vi "Read any file DBL 1ch.vi"(6 "Data type":dbl[](array[numeric]), 7 "tdms file in":refnum<k34>, 8 "error in":errorcluster, 9 "Data File Type":T2(ring), 10 "Data window":T1={"Start"=0, "Length"=500000, "Channel numbers"=[0], "Channel name"="", "Group name"="Untitled"}, 11 "Input file path":path) -> (0 "error out":errorcluster, 1 "1st channel length":u64, 2 "Data out":dbl[](array[numeric]), 3 "Actual input file path":path, 4 "end of file?":bool, 5 "tdms file out":refnum<k34>)   [LabVIEW 2015]
uses:
  Data window.ctl
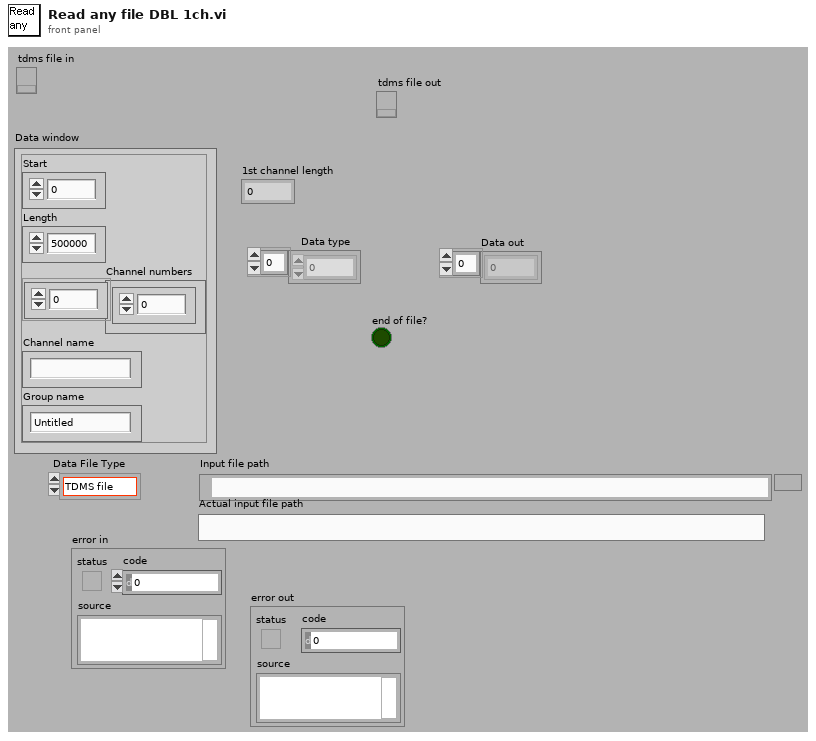
[diagram p1: front panel]
types:
  T1 = typedef "Data window.ctl" = cluster{"Start":i64, "Length":i32, "Channel numbers":i64[], "Channel name":string, "Group name":string}
  T2 = enum16{"TDMS file", "Tektronics ISF", "BinF file", "ASCII File", "BinH File", "BinW File", "BINARY File"}
  T3 = enum16{"open", "open or create", "create or replace", "create", "open (read-only)"}
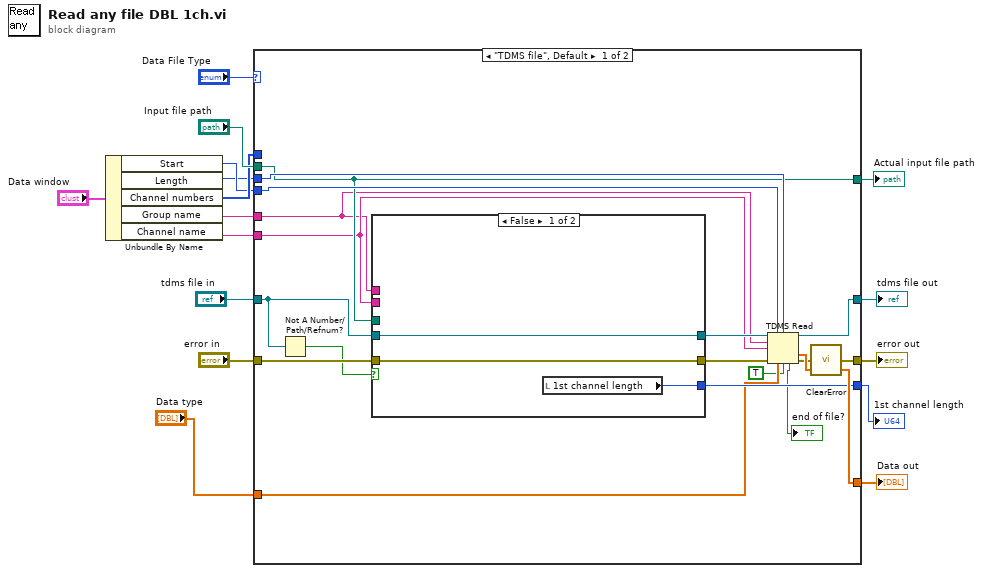
[diagram p0: block diagram]
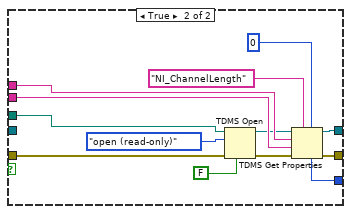
[diagram p2: hidden frame]
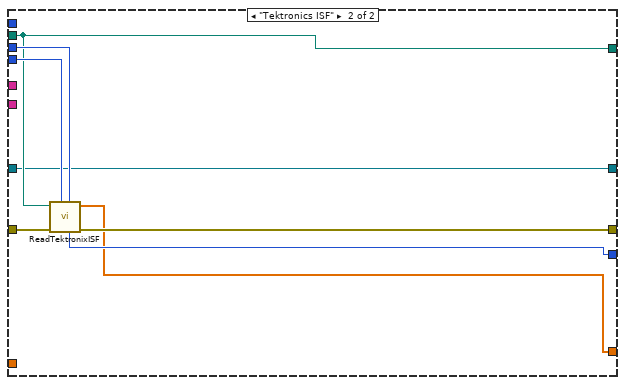
[diagram p3: hidden frame]
diagram:
  n1 = Unbundle By Name("Data window") -> ("Start"=w11:i64, "Length"=w10:i32, "Channel numbers"=w12:i64[], "Group name"=w7:string, "Channel name"=w9:string)
  n2 = case shown="\"TDMS file\", Default" "Data File Type" {
    tunnel: "Input file path" -> [w29 w54]
    tunnel: [w29 w54] -> w14
    tunnel: "error in" -> [w34 w56]
    tunnel: [w24 w55] -> w5
    tunnel: w12 -> [_ _]
    tunnel: w11 -> [w31 w57]
    tunnel: w10 -> [w30 w58]
    tunnel: [w25 w51] -> w2
    tunnel: w9 -> [w22 _]
    tunnel: [w23 w53] -> w8
    tunnel: w7 -> [w21 _]
    tunnel: [w28 w52] -> w4
    tunnel: "tdms file in" -> [w26 w52]
    tunnel: "Data type" -> [w19 _]
    frame "TDMS file", Default {
      n3 = Not A Number/Path/Refnum?(number/path/refnum=w26) -> (NaN/Path/Refnum?=w27:bool)
      n4 = case shown="False" w27 {
        tunnel: w34 -> [w36 w50]
        tunnel: [w37 w39] -> w33
        tunnel: [w36 w44] -> w32
        tunnel: w29 -> [_ w49]
        tunnel: w26 -> [w37 _]
        tunnel: [w35 w43] -> w23
        tunnel: w22 -> [_ w42]
        tunnel: w21 -> [_ w41]
        frame False {
          n5 = local read "1st channel length"() -> (w35:u64)
        }
        frame True {
          n6 = TDMS Open(6:FALSE ("disable buffering (T)"), 8:w50, 10:T3."open (read-only)" ("operation (0:open)"), 11:w49) -> (0:w45:errorcluster, 3:w40:refnum<k34>)  [unwired: 3 in]
          n7 = TDMS Get Properties(5:u64 0, 7:"NI_ChannelLength" ("property name"), 8:w45, 9:w42, 10:w41, 11:w40) -> (0:w44:errorcluster, 3:w39:refnum<k34>, 4:w43:u64)  [unwired: 3 out]
        }
      }
      n8 = TDMS Read(0:w33, 1:w31, 2:w30, 5:w21, 7:w22, 11:w32, 12:w19, 13:TRUE ("return channels in file order? (F)")) -> (4:w28:refnum<k34>, 10:w25:dbl[], 14:→"end of file?":bool, 15:w20:errorcluster)  [unwired: 2 out]
      n9 = call <vilib>:"ClearError.vi"("error in (no error)"=w20) -> ("error out"=w24:errorcluster)
    }
    frame "Tektronics ISF" {
      n10 = call "ReadTektronixISF.vi"("Length"=w58, "Start"=w57, "error in (no error)"=w56, "Path"=w54) -> ("error out"=w55:errorcluster, "Data"=w51:dbl[], "Total number of points"=w53:u64)  [unwired: 5 out]
    }
  }
  "Actual input file path" <- w14
  "error out" <- w5
  "1st channel length" <- w8
  "tdms file out" <- w4
  "Data out" <- w2
